vi "fft_to_linear_between.vi"(1 "Output count":i32=18, 2 "Min frequency":i32, 3 "After FFT":dynamicdata(graph), 4 "Max frequency":i32=24000) -> (0 "After FFT 2":dbl[](array[numeric]))   [LabVIEW 2024]
panel:
  # "18'th"
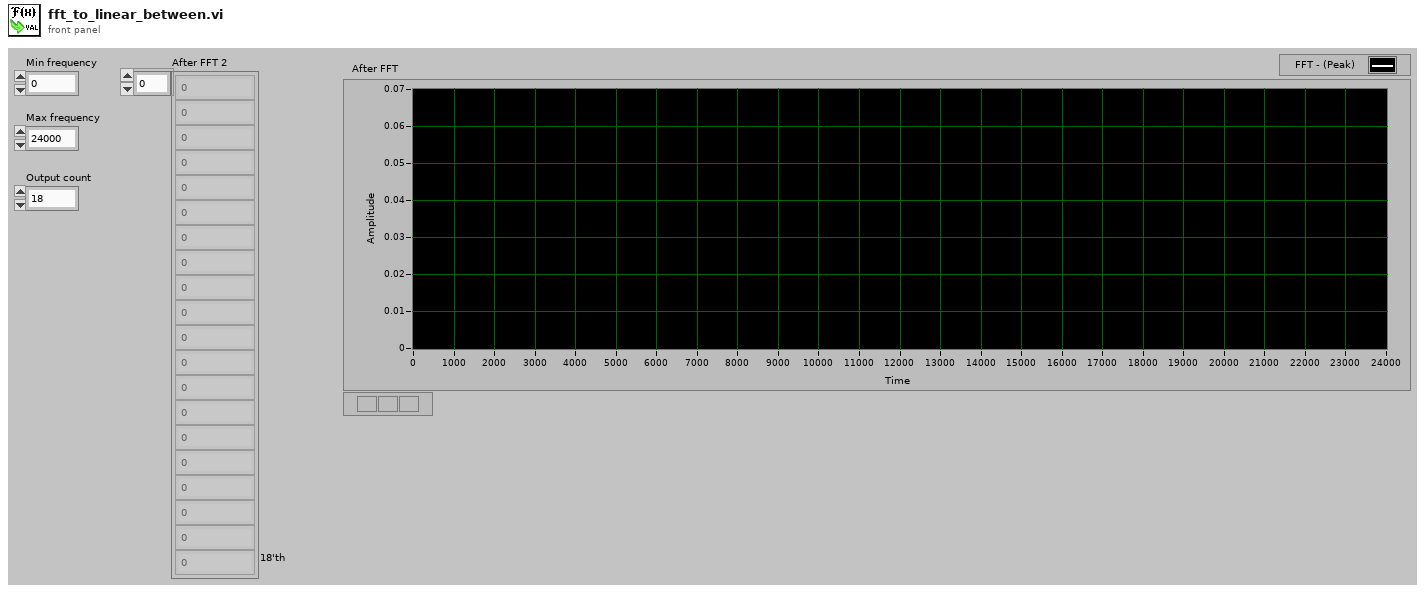
[diagram p1: front panel]
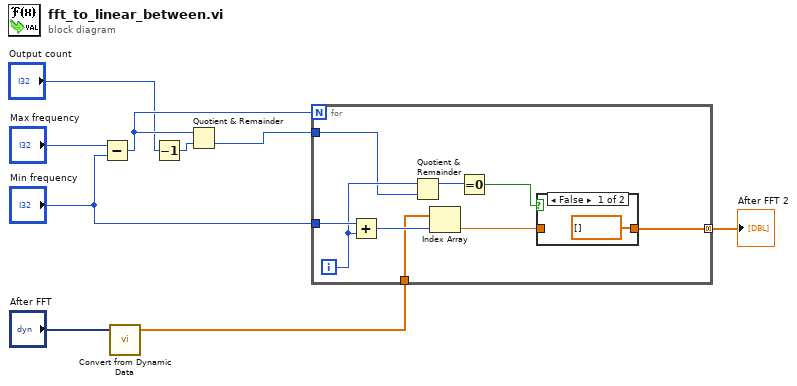
[diagram p0: block diagram]
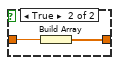
[diagram p2: hidden frame]
diagram:
  n1 = Subtract(x="Max frequency", y="Min frequency") -> (x-y=w5:i32)
  n2 = call "Convert from Dynamic Data"("Dynamic Data Type"="After FFT") -> ("Array"=w3:dbl[])  [unwired: 3 in]
  n3 = Decrement(x="Output count") -> (x-1=w1:i32)
  n4 = Quotient & Remainder(x=w5, y=w1) -> (floor(x/y)=w4:i32)  [unwired: 1 out]
  n5 = for {
    N: w5 -> [_]
    tunnel: w3 -> [w16]
    tunnel: "Min frequency" -> [w17]
    tunnel: [w14] -> w6 mode=concatenating
    tunnel: w4 -> [w12]
    i -> [w13]
    n6 = Add(x=w17, y=w13) -> (x+y=w18:i32)
    n7 = Quotient & Remainder(x=w13, y=w12) -> (x-y*floor(x/y)=w11:i32)  [unwired: 1 out]
    n8 = Index Array(array=w16, index=w18) -> (element=w15:dbl)
    n9 = Equal To 0?(x=w11) -> (x = 0?=w10:bool)
    n10 = case shown="False" w10 {
      tunnel: w15 -> [_ w21]
      tunnel: [dbl[] [] w20] -> w14
      frame False {
      }
      frame True {
        n11 = Build Array(w21) -> (w20:dbl[])
      }
    }
  }
  "After FFT 2" <- w6
